vi "Calculate Sweep Transition Settings.vi"(9 "measurement configuration":T2={"Input channel"=1, "Full scale range"=10.0, "Transition span"=1.5, "Transition step size"=0.05, "Analog source resource name"="", "Digital capture resource name"="", "Digital capture sample rate"=800000.0, "Digital capture samples"=10000, "DMM resource name"="", "DMM range"=10.0, "DMM resolution"=5.5} {"DMM range" format="%#_6pV"; "Digital capture sample rate" format="%#_6pS/s"; "Transition step size" format="%#_gLSB"; "Transition span" format="%#_gLSB"; "Full scale range" format="%#_6pV"}, 10 "Sweep Transition Settings In":T1) -> (2 "Sweep Transition Settings Out":T1)   [LabVIEW 2021, in "adc_fullScaleError.lvlib"]
uses:
  adc_fullScaleError.lvlib
  Measurement Configuration.ctl
  Controls/Sweep Transition Settings.ctl
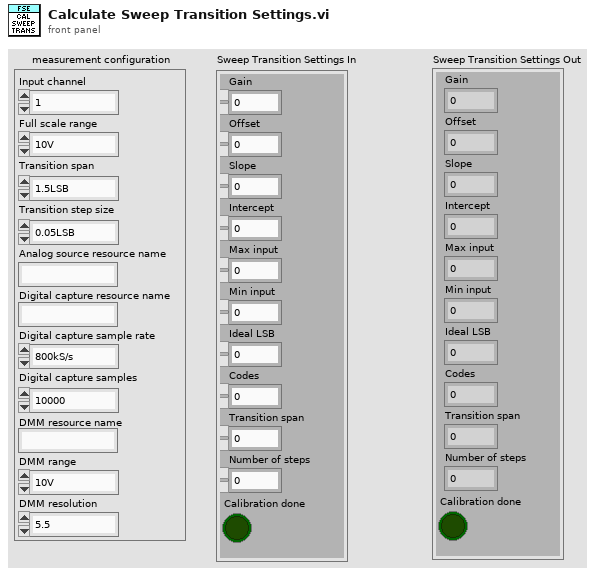
[diagram p1: front panel]
types:
  T1 = typedef "adc_fullScaleError.lvlib/Sweep Transition Settings.ctl" = cluster{"Gain":dbl, "Offset":dbl, "Slope":dbl, "Intercept":dbl, "Max input":dbl, "Min input":dbl, "Ideal LSB":dbl, "Codes":dbl, "Transition span ":dbl, "Number of steps":i32, "Calibration done":bool}
  T2 = typedef "adc_fullScaleError.lvlib/Measurement Configuration.ctl" = cluster{"Input channel":i32, "Full scale range":dbl, "Transition span":dbl, "Transition step size":dbl, "Analog source resource name":string, "Digital capture resource name":string, "Digital capture sample rate":dbl, "Digital capture samples":u32, "DMM resource name":string, "DMM range":dbl, "DMM resolution":dbl}
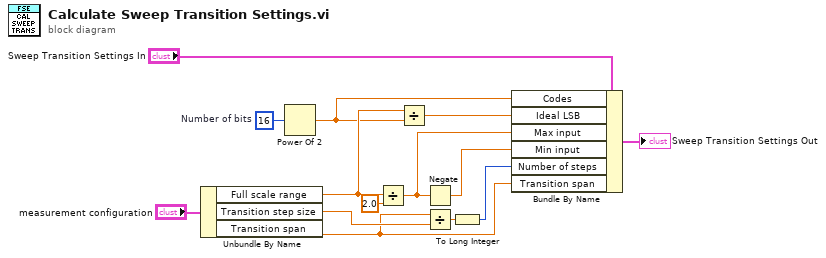
[diagram p0: block diagram]
diagram:
  w3 = i16 16  # Number of bits
  n1 = Unbundle By Name("measurement configuration") -> ("Full scale range"=w12:dbl, "Transition step size"=w11:dbl, "Transition span"=w1:dbl)
  n2 = Power Of 2(x=w3) -> (2^x=w2:dbl)
  n3 = Divide(x=w12, y=2.0) -> (x/y=w7:dbl)
  n4 = Divide(x=w12, y=w2) -> (x/y=w8:dbl)
  n5 = Negate(x=w7) -> (-x=w6:dbl)
  n6 = Divide(x=w1, y=w11) -> (x/y=w10:dbl)
  n7 = To Long Integer(number=w10) -> (32bit integer=w5:i32)
  n8 = Bundle By Name(cluster="Sweep Transition Settings In", "Codes"=w2, "Ideal LSB"=w8, "Max input"=w7, "Min input"=w6, "Number of steps"=w5, "Transition span"=w1) -> (→"Sweep Transition Settings Out":T1)
